vi "newRegionTester.vi"() -> ()   [LabVIEW 2013]
panel:
  in  "Down":bool
  in  "Up":bool
  in  "UpLimit":bool
  in  "DownLimit":bool
  out "Motor Output":dbl
  out "Region":dbl
  in  "Up2":bool
  in  "Center":bool
  in  "Down2":bool
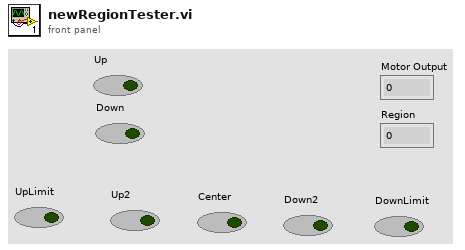
[diagram p1: front panel]
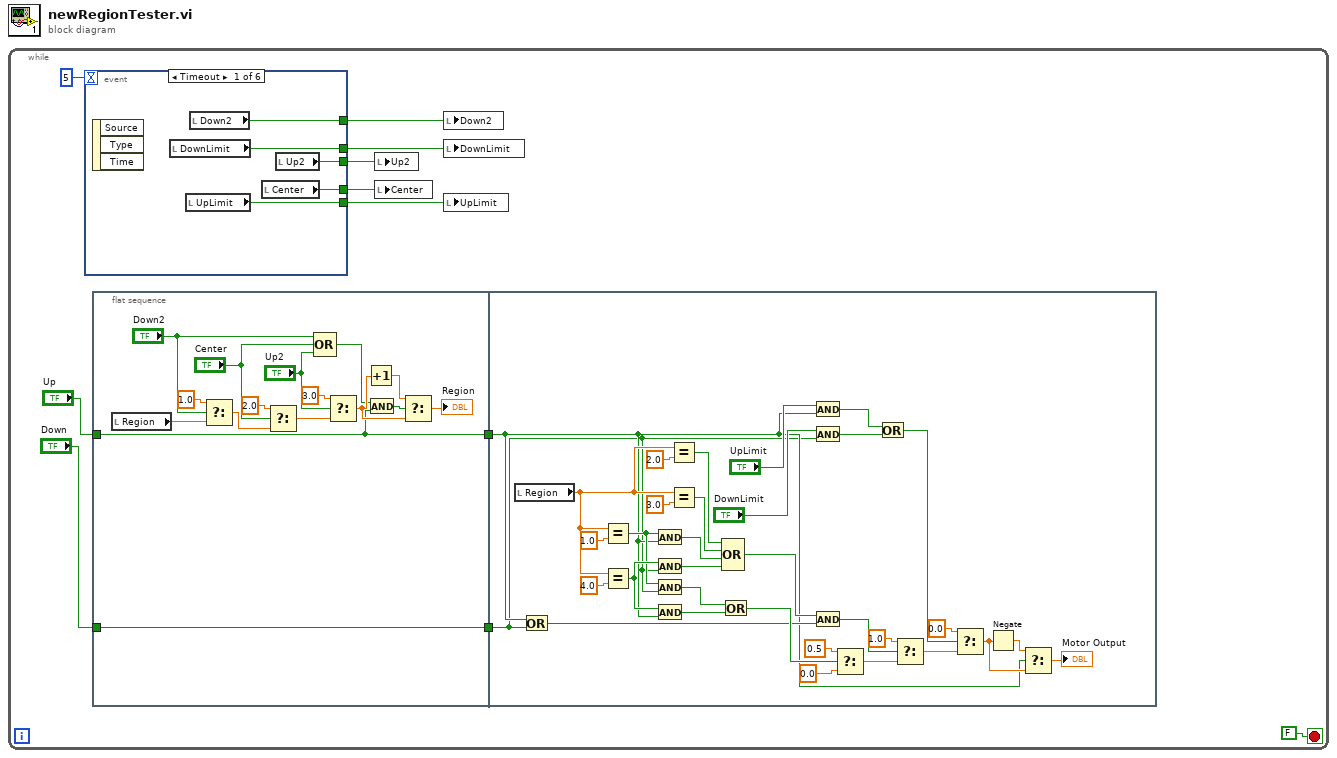
[diagram p0: block diagram]
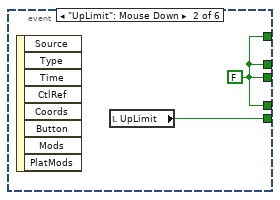
[diagram p2: hidden frame]
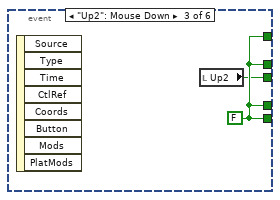
[diagram p3: hidden frame]
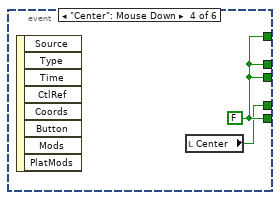
[diagram p4: hidden frame]
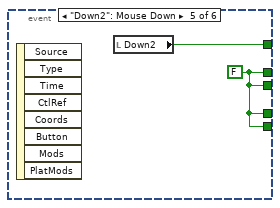
[diagram p5: hidden frame]
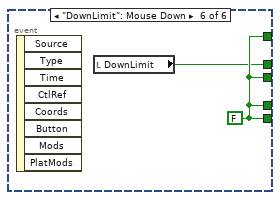
[diagram p6: hidden frame]
diagram:
  n1 = while {
    stop <- FALSE stop-if-true
    n2 = event shown="[0] Timeout" {
      selector: _ -> [_ _ _ _ _ _]
      dyn-events: _ -> [_ _ _ _ _ _]
      timeout: 5 -> [_ _ _ _ _ _]
      tunnel: [w16 w17 w20 w22 w24 w26] -> w9
      tunnel: [w13 w18 w19 w22 w24 w26] -> w8
      tunnel: [w12 w18 w20 w21 w24 w26] -> w7
      tunnel: [w15 w18 w20 w22 w23 w26] -> w6
      tunnel: [w14 w18 w20 w22 w24 w25] -> w5
      event Timeout {
        n3 = event-data() -> ()  [unwired: 1 in, 3 out]
        n4 = local read "DownLimit"() -> (w14:bool)
        n5 = local read "UpLimit"() -> (w16:bool)
        n6 = local read "Down2"() -> (w15:bool)
        n7 = local read "Center"() -> (w12:bool)
        n8 = local read "Up2"() -> (w13:bool)
      }
      event "UpLimit": Mouse Down {
        w18 = FALSE
        n9 = event-data() -> ()  [unwired: 1 in, 8 out]
        n10 = local read "UpLimit"() -> (w17:bool)
      }
      event "Up2": Mouse Down {
        w20 = FALSE
        n11 = event-data() -> ()  [unwired: 1 in, 8 out]
        n12 = local read "Up2"() -> (w19:bool)
      }
      event "Center": Mouse Down {
        w22 = FALSE
        n13 = event-data() -> ()  [unwired: 1 in, 8 out]
        n14 = local read "Center"() -> (w21:bool)
      }
      event "Down2": Mouse Down {
        w24 = FALSE
        n15 = event-data() -> ()  [unwired: 1 in, 8 out]
        n16 = local read "Down2"() -> (w23:bool)
      }
      event "DownLimit": Mouse Down {
        w26 = FALSE
        n17 = event-data() -> ()  [unwired: 1 in, 8 out]
        n18 = local read "DownLimit"() -> (w25:bool)
      }
    }
    n19 = flat-sequence {
      tunnel: "Down" -> [w33]
      tunnel: [w33] -> w3
      tunnel: [w28] -> w2
      tunnel: "Up" -> [w28]
      tunnel: w3 -> [w44]
      tunnel: w2 -> [w45]
      frame #0 {
        n20 = local read "Region"() -> (w42:dbl)
        n21 = Select(t=1.0, s="Down2", f=w42) -> (s? t:f=w37:dbl)
        n22 = Select(t=2.0, s="Center", f=w37) -> (s? t:f=w38:dbl)
        n23 = Compound Arithmetic op=OR("Down2", "Center", "Up2") -> (w29:bool)
        n24 = Select(t=3.0, s="Up2", f=w38) -> (s? t:f=w39:dbl)
        n25 = Increment(x=w39) -> (x+1=w40:dbl)
        n26 = And(x=w29, y=w28) -> (x .and. y?=w27:bool)
        n27 = Select(t=w40, s=w27, f=w39) -> (s? t:f=→"Region":dbl)
      }
      frame #1 {
        n28 = local read "Region"() -> (w72:dbl)
        n29 = Or(x=w45, y=w44) -> (x .or. y?=w46:bool)
        n30 = Equal?(x=w72, y=1.0) -> (x = y?=w59:bool)
        n31 = Equal?(x=w72, y=4.0) -> (x = y?=w60:bool)
        n32 = And(x=w59, y=w45) -> (x .and. y?=w52:bool)
        n33 = And(x=w60, y=w44) -> (x .and. y?=w53:bool)
        n34 = And(x=w59, y=w44) -> (x .and. y?=w58:bool)
        n35 = And(x=w60, y=w45) -> (x .and. y?=w57:bool)
        n36 = Equal?(x=w72, y=2.0) -> (x = y?=w48:bool)
        n37 = Equal?(x=w72, y=3.0) -> (x = y?=w50:bool)
        n38 = Or(x=w58, y=w57) -> (x .or. y?=w61:bool)
        n39 = Compound Arithmetic op=OR(w48, w50, w52, w53) -> (w47:bool)
        n40 = And(x="UpLimit", y=w45) -> (x .and. y?=w64:bool)
        n41 = And(x="DownLimit", y=w44) -> (x .and. y?=w65:bool)
        n42 = And(x=w47, y=w46) -> (x .and. y?=w43:bool)
        n43 = Select(t=0.5, s=w61, f=0.0) -> (s? t:f=w63:dbl)
        n44 = Or(x=w64, y=w65) -> (x .or. y?=w66:bool)
        n45 = Select(t=1.0, s=w43, f=w63) -> (s? t:f=w69:dbl)
        n46 = Select(t=0.0, s=w66, f=w69) -> (s? t:f=w71:dbl)
        n47 = Negate(x=w71) -> (-x=w70:dbl)
        n48 = Select(t=w70, s=w45, f=w71) -> (s? t:f=→"Motor Output":dbl)
      }
    }
    n49 = local write "Up2"(w8) -> ()
    n50 = local write "Center"(w7) -> ()
    n51 = local write "Down2"(w6) -> ()
    n52 = local write "DownLimit"(w5) -> ()
    n53 = local write "UpLimit"(w9) -> ()
  }
